vi "M08 TV.vi"(11 "NXT/EV3":T1) -> (3 "EV3 out":T1)   [LabVIEW 2016]
uses:
  <vilib>/NXT/Subs/LVHSConnector.ctl
  <vilib>/NXT/LegoClasses/BrickReference/BrickReference.lvclass
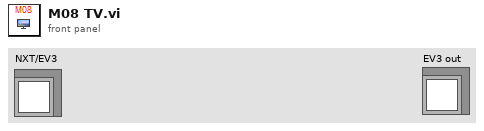
[diagram p1: front panel]
types:
  T1 = typedef "LVHSConnector.ctl" = refnum<class "BrickReference.lvclass">
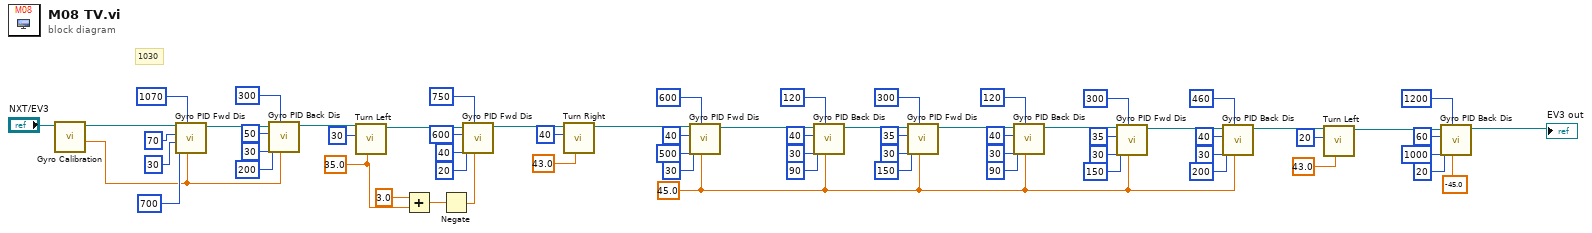
[diagram p0: block diagram]
diagram:
  w10 = sgl 45.0 ("Target angle")
  w48 = sgl 35.0 ("Turning angle")
  # "1030"
  n1 = call "Gyro Calibration.vi"("NXT/EV3"="NXT/EV3") -> ("Degrees"=w56:sgl, "NXT/EV3"=w67:T1)  [unwired: 6 in, 1 out]
  n2 = call "Gyro PID Fwd Dis.vi"("Target angle"=w56, "Threshold to stop"=1070, "Threshold to slow"=700, "Min. speed"=30, "Max. speed"=70, "EV3 in"=w67) -> ("EV3 out"=w61:T1)  [unwired: 5 in]
  n3 = call "Gyro PID Back Dis.vi"("Target angle"=w56, "Threshold to stop"=300, "Threshold to slow"=200, "Min. speed"=30, "Max. speed"=50, "EV3 in"=w61) -> ("EV3 out"=w55:T1)  [unwired: 5 in]
  n4 = call "Turn Left.vi"("Turning angle"=w48, "Motor B (right)"=i8 30, "EV3 in"=w55) -> ("EV3 out"=w53:T1)  [unwired: 8 in]
  n5 = Add(x=sgl 3.0, y=w48) -> (x+y=w46:sgl)
  n6 = Negate(x=w46) -> (-x=w45:sgl)
  n7 = call "Gyro PID Fwd Dis.vi"("Target angle"=w45, "Threshold to stop"=750, "Threshold to slow"=20, "Min. speed"=40, "Max. speed"=600, "EV3 in"=w53) -> ("EV3 out"=w44:T1)  [unwired: 5 in]
  n8 = call "Turn Right.vi"("Turning angle"=sgl 43.0, "Motor B (right)"=i8 40, "EV3 in"=w44) -> ("EV3 out"=w41:T1)  [unwired: 8 in]
  n9 = call "Gyro PID Fwd Dis.vi"("Target angle"=w10, "Threshold to stop"=600, "Threshold to slow"=30, "Min. speed"=500, "Max. speed"=40, "EV3 in"=w41) -> ("EV3 out"=w36:T1)  [unwired: 5 in]
  n10 = call "Gyro PID Back Dis.vi"("Target angle"=w10, "Threshold to stop"=120, "Threshold to slow"=90, "Min. speed"=30, "Max. speed"=40, "EV3 in"=w36) -> ("EV3 out"=w31:T1)  [unwired: 5 in]
  n11 = call "Gyro PID Fwd Dis.vi"("Target angle"=w10, "Threshold to stop"=300, "Threshold to slow"=150, "Min. speed"=30, "Max. speed"=35, "EV3 in"=w31) -> ("EV3 out"=w26:T1)  [unwired: 5 in]
  n12 = call "Gyro PID Back Dis.vi"("Target angle"=w10, "Threshold to stop"=120, "Threshold to slow"=90, "Min. speed"=30, "Max. speed"=40, "EV3 in"=w26) -> ("EV3 out"=w20:T1)  [unwired: 5 in]
  n13 = call "Gyro PID Fwd Dis.vi"("Target angle"=w10, "Threshold to stop"=300, "Threshold to slow"=150, "Min. speed"=30, "Max. speed"=35, "EV3 in"=w20) -> ("EV3 out"=w16:T1)  [unwired: 5 in]
  n14 = call "Gyro PID Back Dis.vi"("Target angle"=w10, "Threshold to stop"=460, "Threshold to slow"=200, "Min. speed"=30, "Max. speed"=40, "EV3 in"=w16) -> ("EV3 out"=w11:T1)  [unwired: 5 in]
  n15 = call "Turn Left.vi"("Turning angle"=sgl 43.0, "Motor B (right)"=i8 20, "EV3 in"=w11) -> ("EV3 out"=w7:T1)  [unwired: 8 in]
  n16 = call "Gyro PID Back Dis.vi"("Target angle"=sgl -45.0, "Threshold to stop"=1200, "Threshold to slow"=20, "Min. speed"=1000, "Max. speed"=60, "EV3 in"=w7) -> ("EV3 out"=→"EV3 out":T1)  [unwired: 5 in]
